vi "GetDSCValues.vi"() -> (3 "cluster":T1)   [LabVIEW 2016]
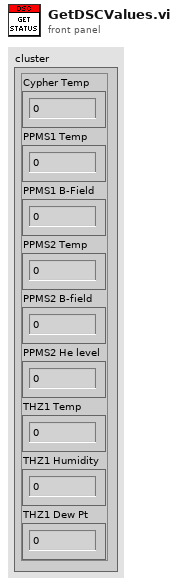
[diagram p1: front panel]
types:
  T1 = cluster{"Cypher Temp":dbl, "PPMS1 Temp":dbl, "PPMS1 B-Field":dbl, "PPMS2 Temp":dbl, "PPMS2 B-field":dbl, "PPMS2 He level":dbl, "THZ1 Temp":dbl, "THZ1 Humidity":dbl, "THZ1 Dew Pt":dbl}
  T2 = cluster{"shared variable refnum in":refnum<k21>, "shared variable refnum in 2":refnum<k21>, "shared variable refnum in 3":refnum<k21>, "shared variable refnum in 4":refnum<k21>, "shared variable refnum in 5":refnum<k21>, "shared variable refnum in 6":refnum<k21>, "shared variable refnum in 7":refnum<k21>, "shared variable refnum in 8":refnum<k21>, "shared variable refnum in 9":refnum<k21>, "shared variable refnum in 10":refnum<k21>}
  T3 = cluster{"[0]":dbl, "[1]":dbl, "[2]":dbl, "[3]":dbl, "[4]":dbl, "[5]":dbl, "[6]":dbl, "[7]":dbl, "[8]":dbl}
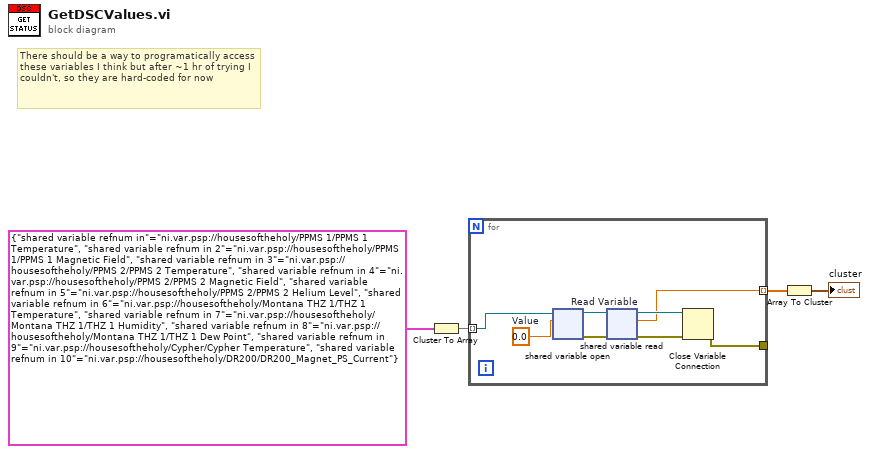
[diagram p0: block diagram]
diagram:
  # "There should be a way to programatically access these variables I think but after ~1 hr of trying I couldn't, so they are hard-coded for now"
  n1 = Cluster To Array(cluster=T2 {"shared variable refnum in"="ni.var.psp://housesoftheholy/PPMS 1/PPMS 1 Temperature", "shared variable refnum in 2"="ni.var.psp://housesoftheholy/PPMS 1/PPMS 1 Magnetic Field", "shared variable refnum in 3"="ni.var.psp://housesoftheholy/PPMS 2/PPMS 2 Temperature", "shared variable refnum in 4"="ni.var.psp://housesoftheholy/PPMS 2/PPMS 2 Magnetic Field", "shared variable refnum in 5"="ni.var.psp://housesoftheholy/PPMS 2/PPMS 2 Helium Level", "shared variable refnum in 6"="ni.var.psp://housesoftheholy/Montana THZ 1/THZ 1 Temperature", "shared variable refnum in 7"="ni.var.psp://housesoftheholy/Montana THZ 1/THZ 1 Humidity", "shared variable refnum in 8"="ni.var.psp://housesoftheholy/Montana THZ 1/THZ 1 Dew Point", "shared variable refnum in 9"="ni.var.psp://housesoftheholy/Cypher/Cypher Temperature", "shared variable refnum in 10"="ni.var.psp://housesoftheholy/DR200/DR200_Magnet_PS_Current"}) -> (array=w3:refnum<k21>[])
  n2 = for {
    tunnel: [w7] -> _
    tunnel: w3 -> [w8] mode=indexing
    tunnel: [w5] -> w1 mode=indexing
    w9 = 0.0  # Value
    n3 = shared-variable-open(w8, w9) -> (w12:refnum<k21>, w10:errorcluster)  [unwired: 1 in]
    n4 = shared-variable-read "Read Variable"(w12, w10) -> (w11:refnum<k21>, w6:errorcluster, w5:dbl)  [unwired: 1 out]
    n5 = Close Variable Connection(8:w6, 11:w11) -> (0:w7:errorcluster)
  }
  n6 = Array To Cluster(array=w1) -> (cluster=→"cluster":T3)
